vi "ReserveRobot.vi"(0 "Universal Robot.lvclass in":refnum<class "Universal Robot.lvclass">, 5 "error in (no error)":errorcluster) -> (14 "Universal Robot.lvclass out":refnum<class "Universal Robot.lvclass">, 19 "error out":errorcluster)   [LabVIEW 2019, in "Universal Robot.lvclass"]
uses:
  Universal Robot.lvclass
  Universal Robot.lvclass/Universal Robot.ctl
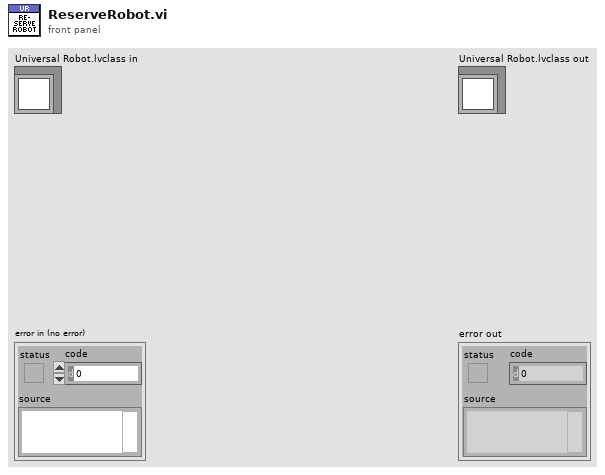
[diagram p1: front panel]
types:
  T1 = typedef "Semaphore RefNum" = refnum<k1>
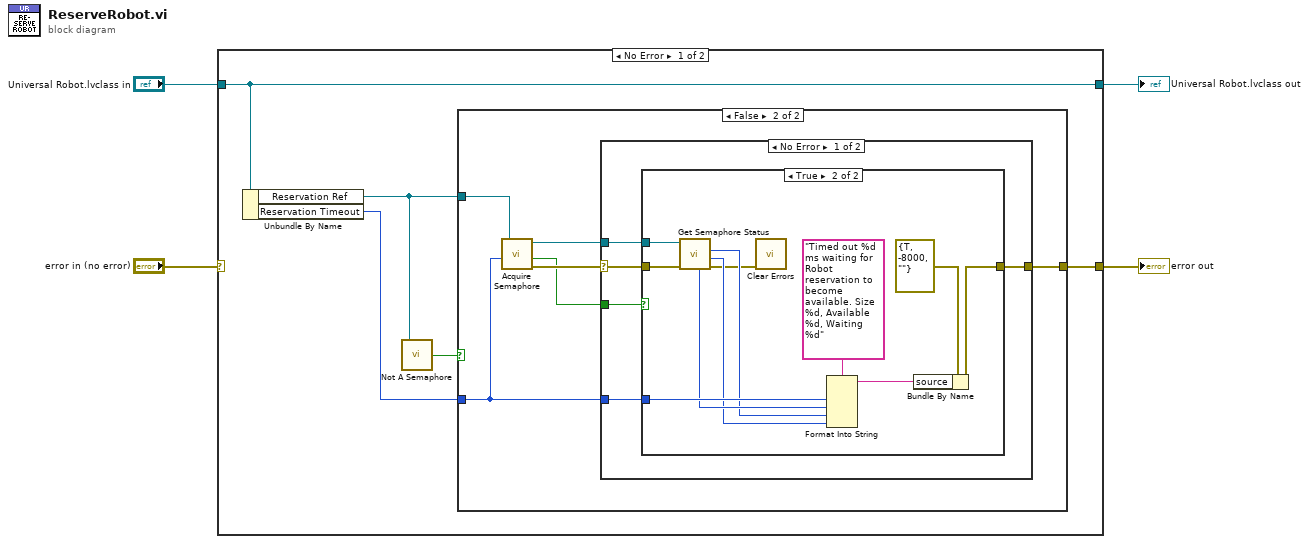
[diagram p0: block diagram]
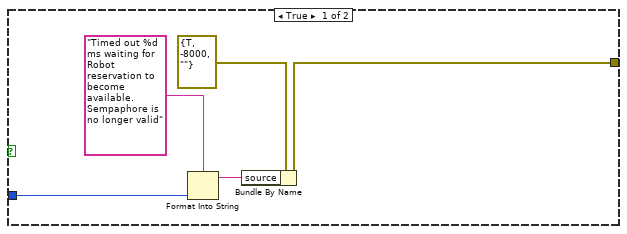
[diagram p2: hidden frame]
diagram:
  n1 = case shown="No Error" "error in (no error)" {
    selector: "error in (no error)" -> [_ w40]
    tunnel: [w8 w40] -> w3
    tunnel: [w5 w39] -> w1
    tunnel: "Universal Robot.lvclass in" -> [w5 w39]
    frame No Error {
      n2 = Unbundle By Name(w5) -> ("Reservation Ref"=w7:T1, "Reservation Timeout"=w9:i32)
      n3 = call <vilib>:"Not A Semaphore.vi"("semaphore"=w7) -> ("not a semaphore"=w6:bool)
      n4 = case shown="False" w6 {
        tunnel: w9 -> [w14 w17]
        tunnel: [w13 w16] -> w8
        tunnel: w7 -> [_ w15]
        frame True {
          n5 = Format Into String(format string="Timed out %d ms waiting for Robot reservation to become available. Sempaphore is no longer valid" ("source"), w14) -> (resulting string=w12:string)  [unwired: 2 in, 1 out]
          n6 = Bundle By Name(cluster=errorcluster {"status"=TRUE, "code"=-8000, "source"=""} ("error constant"), "source"=w12) -> (w13:errorcluster)
        }
        frame False {
          n7 = call <vilib>:"Acquire Semaphore.vi"("ms timeout (-1)"=w17, "semaphore"=w15) -> ("error out"=w20:errorcluster, "timed out"=w19:bool, "semaphore out"=w18:T1)  [unwired: 3 in]
          n8 = case shown="No Error" w20 {
            selector: w20 -> [w23 w38]
            tunnel: w19 -> [w25 _]
            tunnel: w18 -> [w24 _]
            tunnel: [w22 w38] -> w16
            tunnel: w17 -> [w21 _]
            frame No Error {
              n9 = case shown="True" w25 {
                tunnel: w24 -> [_ w37]
                tunnel: w23 -> [w26 w27]
                tunnel: [w26 w35] -> w22
                tunnel: w21 -> [_ w36]
                frame False {
                }
                frame True {
                  n10 = call <vilib>:"Get Semaphore Status.vi"("error in (no error)"=w27, "semaphore"=w37) -> ("error out"=w28:errorcluster, "# waiting"=w30:i32, "# available"=w29:i32, "size"=w31:i32)  [unwired: 4 in, 2 out]
                  n11 = call <vilib>:"Clear Errors.vi"("error in (no error)"=w28) -> ()  [unwired: 5 in, 2 out]
                  n12 = Format Into String(format string="Timed out %d ms waiting for Robot reservation to become available. Size %d, Available %d, Waiting %d" ("source"), w36, w31, w29, w30) -> (resulting string=w34:string)  [unwired: 2 in, 1 out]
                  n13 = Bundle By Name(cluster=errorcluster {"status"=TRUE, "code"=-8000, "source"=""} ("error constant"), "source"=w34) -> (w35:errorcluster)
                }
              }
            }
            frame Error {
            }
          }
        }
      }
    }
    frame Error {
    }
  }
  "error out" <- w3
  "Universal Robot.lvclass out" <- w1
